vi "Remove Channel.vi"() -> ()   [LabVIEW 2011, in "IVI DC Power Supply Custom Device.lvlib"]
uses:
  IVI DC Power Supply Custom Device.lvlib
  <vilib>/NI Veristand/Custom Device API/Custom Device Item Ref.ctl
  <vilib>/NI Veristand/Custom Device API/Custom Device API.lvlib
panel:
  out "error out":errorcluster
  in  "error in (no error)":errorcluster
  in  "Node Ptr":T1 format="%.0x"
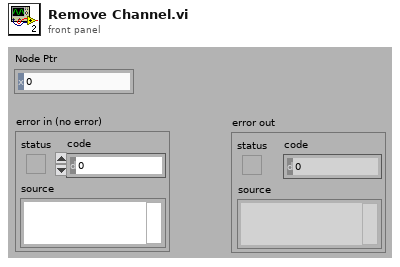
[diagram p1: front panel]
types:
  T1 = typedef "Custom Device API.lvlib/Custom Device Item Ref.ctl" = u64
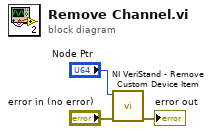
[diagram p0: block diagram]
diagram:
  n1 = call <vilib>:"NI VeriStand - Remove Custom Device Item.vi"("error in (no error)"="error in (no error)", "Item Ref in"="Node Ptr") -> ("error out"=→"error out":errorcluster)  [unwired: 8 in, 1 out]
